vi "get_predictions.vi"(1 "2D array":dbl[][](array[numeric])) -> (0 "Array":i32[](array[numeric]))   [LabVIEW 2023]
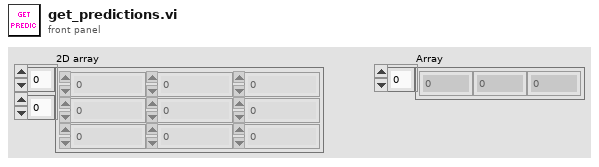
[diagram p1: front panel]
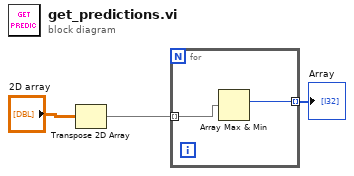
[diagram p0: block diagram]
diagram:
  n1 = Transpose 2D Array(2D array="2D array") -> (transposed array=w2:dbl[][])
  n2 = for {
    tunnel: w2 -> [w5] mode=indexing
    tunnel: [w4] -> w3 mode=indexing
    n3 = Array Max & Min(array=w5) -> (max index (indices)=w4:i32)  [unwired: 3 out]
  }
  "Array" <- w3
